vi "Calibrate VNA.vi"(8 "error in (no error)":errorcluster, 9 "Cal kit type":enum16{"E-CAL", "Mechanical"}(ring), 10 "Calibration mode":enum16{"1 Port", "2  Port", "3 Port", "4 Port"}(ring), 11 "VNA-PNA in":refnum<class "VNA-PNA.lvclass">) -> (0 "error out":errorcluster, 3 "VNA-PNA out":refnum<class "VNA-PNA.lvclass">)   [LabVIEW 2020, in "VNA-PNA.lvclass"]
uses:
  VNA-PNA.lvclass
  C:/Sandbox/Git_Sandbox/WiSpry Test Framework source code (LV20)/WiSpry Test Framework/Instruments/Instrument.lvclass
  C:/Sandbox/Git_Sandbox/WiSpry Test Framework source code (LV20)/WiSpry Test Framework/Instruments/Vector Network Analyzer/Vector Network Analyzer.lvclass
  Vector Network Analyzer.lvclass/Vector Network Analyzer.ctl
  Instrument.lvclass/Instrument.ctl
  Instrument.lvclass
  Vector Network Analyzer.lvclass
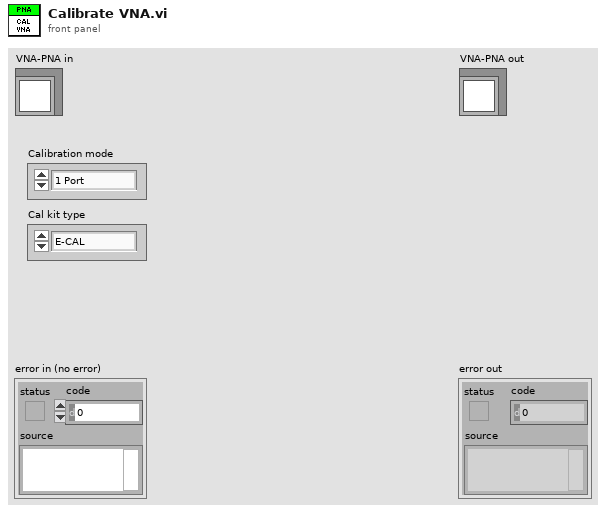
[diagram p1: front panel]
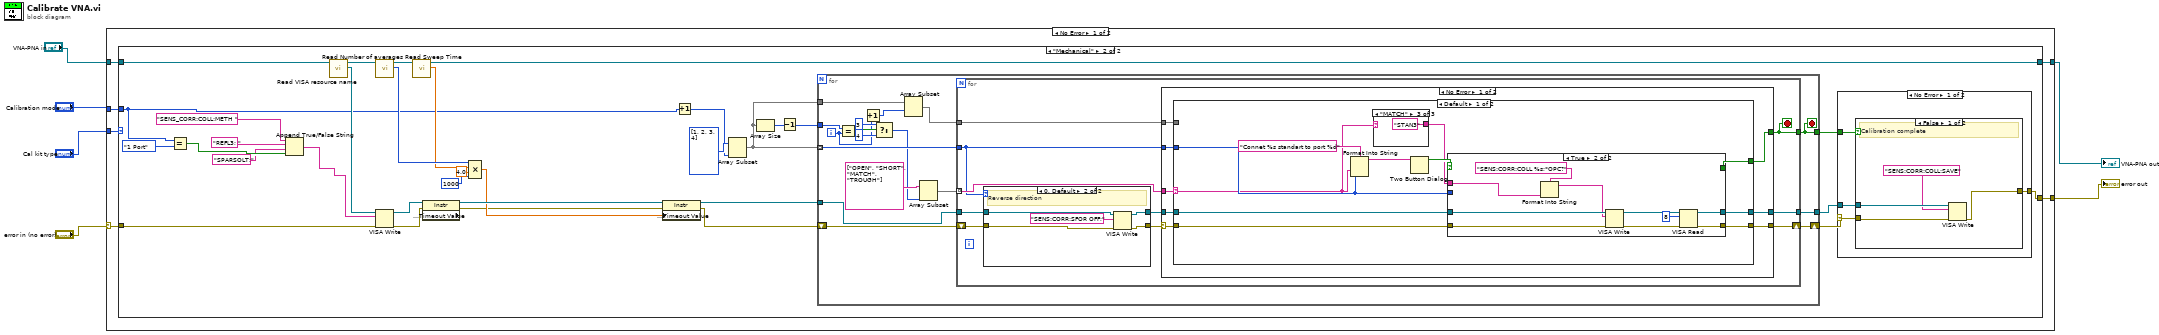
[diagram p0: block diagram]
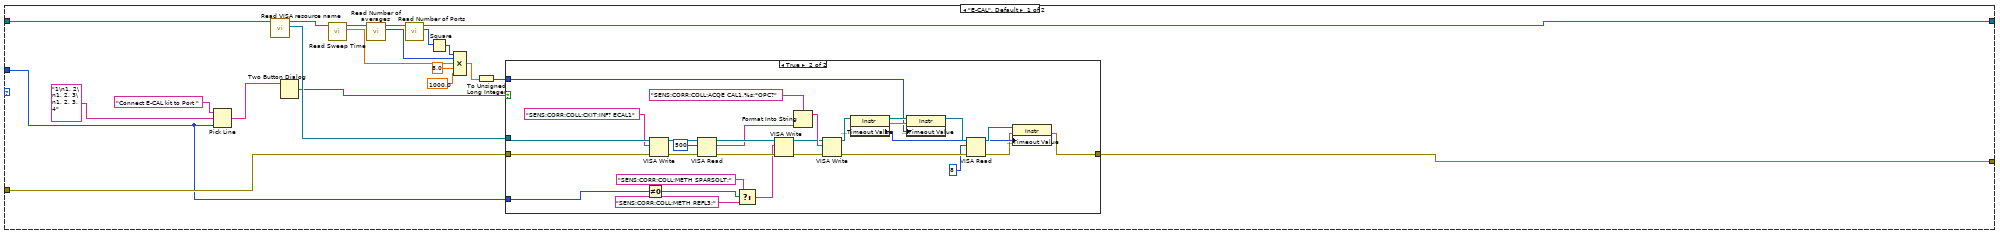
[diagram p2: hidden frame]
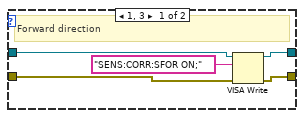
[diagram p6: hidden frame]
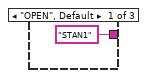
[diagram p7: hidden frame]
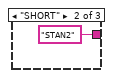
[diagram p8: hidden frame]
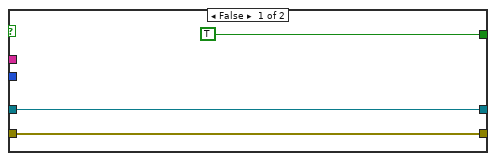
[diagram p9: hidden frame]
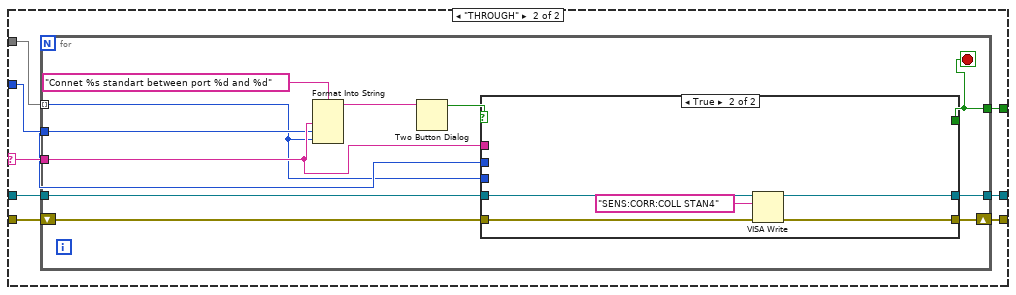
[diagram p10: hidden frame]
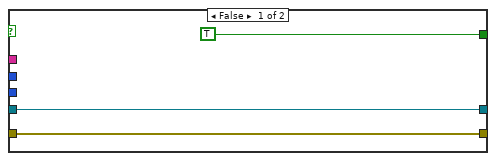
[diagram p11: hidden frame]
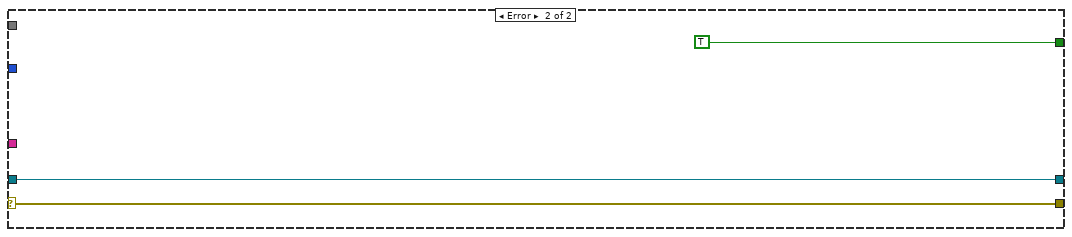
[diagram p12: hidden frame]
diagram:
  n1 = case shown="No Error" "error in (no error)" {
    selector: "error in (no error)" -> [w10 w209]
    tunnel: "Calibration mode" -> [w12 _]
    tunnel: "VNA-PNA in" -> [w11 w210]
    tunnel: [w9 w209] -> w3
    tunnel: [w8 w210] -> w2
    tunnel: "Cal kit type" -> [w7 _]
    frame No Error {
      n2 = case shown="\"Mechanical\"" w7 {
        tunnel: w12 -> [w13 w66]
        tunnel: w11 -> [w33 w91]
        tunnel: w10 -> [w31 w92]
        tunnel: [w30 w67] -> w9
        tunnel: [w23 w73] -> w8
        frame "E-CAL", Default {
          n3 = Pick Line(string ("")="Connect E-CAL kit to Port " ("message"), multi-line string="1\n1, 2\n1, 2, 3\n1, 2, 3, 4", line index=w13) -> (output string=w26:string)
          n4 = call "Read VISA resource name.vi"("Instrument in"=w33) -> ("VISA resource name"=w32:refnum<visa-resource-name>, "Instrument out"=w25:refnum<class "VNA-PNA.lvclass">)  [unwired: 9 in]
          n5 = Two Button Dialog(message=w26) -> (T button?=w29:bool)  [unwired: 2 in]
          n6 = call "Read Sweep Time.vi"("Vector Network Analyzer in"=w25) -> ("Sweep Time"=w18:dbl, "Vector Network Analyzer out"=w24:refnum<class "VNA-PNA.lvclass">)  [unwired: 9 in]
          n7 = call "Read Number of averages.vi"("Vector Network Analyzer in"=w24) -> ("Number of averages"=w19:i32, "Vector Network Analyzer out"=w22:refnum<class "VNA-PNA.lvclass">)  [unwired: 9 in]
          n8 = call "Read Number of Ports.vi"("Vector Network Analyzer in"=w22) -> ("Number of Ports"=w21:i32, "Vector Network Analyzer out"=w23:refnum<class "VNA-PNA.lvclass">)  [unwired: 9 in]
          n9 = Square(x=w21) -> (x^2=w20:i32)
          n10 = Compound Arithmetic op=MULTIPLY(w20, w19, w18, 8.0 ("value"), 1000.0 ("value")) -> (w15:dbl)
          n11 = To Unsigned Long Integer(number=w15) -> (unsigned 32bit integer=w14:u32)
          n12 = case shown="True" w29 {
            tunnel: w32 -> [_ w51]
            tunnel: w31 -> [w34 w52]
            tunnel: [w34 w53] -> w30
            tunnel: w14 -> [_ w54]
            tunnel: w13 -> [_ w44]
            frame False {
            }
            frame True {
              n13 = Not Equal To 0?(x=w44) -> (x != 0?=w43:bool)
              n14 = VISA Write(VISA resource name=w51, write buffer="SENS:CORR:COLL:CKIT:INF? ECAL1", error in (no error)=w52) -> (VISA resource name out=w48:refnum<visa-resource-name>, error out=w49:errorcluster)  [unwired: 1 out]
              n15 = VISA Read(VISA resource name=w48, byte count=u32 500, error in (no error)=w49) -> (VISA resource name out=w46:refnum<visa-resource-name>, read buffer=w38:string, error out=w45:errorcluster)  [unwired: 1 out]
              n16 = Select(t="SENS:CORR:COLL:METH SPARSOLT;" ("write buffer"), s=w43, f="SENS:CORR:COLL:METH REFL3;") -> (s? t:f=w41:string)
              n17 = VISA Write(VISA resource name=w46, write buffer=w41, error in (no error)=w45) -> (VISA resource name out=w36:refnum<visa-resource-name>, error out=w35:errorcluster)  [unwired: 1 out]
              n18 = Format Into String(format string="SENS:CORR:COLL:ACQE CAL1,%s;*OPC?", w38) -> (resulting string=w37:string)  [unwired: 2 in, 1 out]
              n19 = VISA Write(VISA resource name=w36, write buffer=w37, error in (no error)=w35) -> (VISA resource name out=w63:refnum<visa-resource-name>, error out=w59:errorcluster)  [unwired: 1 out]
              n20 = property class="Instr"(reference=w63) -> (reference out=w62:refnum<visa-resource-name>, error out=w61:errorcluster, "General Settings:Timeout Value"=w56:u32)  [unwired: 1 in]
              n21 = property class="Instr"(reference=w62, error in=w61, "General Settings:Timeout Value"=w54) -> (reference out=w60:refnum<visa-resource-name>)  [unwired: 1 out]
              n22 = VISA Read(VISA resource name=w60, byte count=u32 8, error in (no error)=w59) -> (VISA resource name out=w57:refnum<visa-resource-name>, error out=w55:errorcluster)  [unwired: 2 out]
              n23 = property class="Instr"(reference=w57, error in=w55, "General Settings:Timeout Value"=w56) -> (error out=w53:errorcluster)  [unwired: 1 out]
            }
          }
        }
        frame "Mechanical" {
          n24 = Equal?(x=w66, y=enum16{"1 Port", "2  Port", "3 Port", "4 Port"}."1 Port") -> (x = y?=w95:bool)
          n25 = Append True/False String(1:w95, 2:"SPARSOLT;", 3:"REFL3; ", 4:"SENS_CORR:COLL:METH ") -> (0:w65:string)
          n26 = call "Read VISA resource name.vi"("Instrument in"=w91) -> ("VISA resource name"=w90:refnum<visa-resource-name>, "Instrument out"=w85:refnum<class "VNA-PNA.lvclass">)  [unwired: 9 in]
          n27 = call "Read Number of averages.vi"("Vector Network Analyzer in"=w85) -> ("Number of averages"=w83:i32, "Vector Network Analyzer out"=w84:refnum<class "VNA-PNA.lvclass">)  [unwired: 9 in]
          n28 = VISA Write(VISA resource name=w90, write buffer=w65, error in (no error)=w92) -> (VISA resource name out=w81:refnum<visa-resource-name>, error out=w80:errorcluster)  [unwired: 1 out]
          n29 = call "Read Sweep Time.vi"("Vector Network Analyzer in"=w84) -> ("Sweep Time"=w82:dbl, "Vector Network Analyzer out"=w73:refnum<class "VNA-PNA.lvclass">)  [unwired: 9 in]
          n30 = property class="Instr" props=["General Settings:Timeout Value"](reference=w81, error in=w80) -> (reference out=w79:refnum<visa-resource-name>, error out=w76:errorcluster)  [unwired: 1 out]
          n31 = Compound Arithmetic op=MULTIPLY(w83, w82, 4.0 ("value"), 1000 ("value")) -> (w77:dbl)
          n32 = property class="Instr"(reference=w79, error in=w76, "General Settings:Timeout Value"=w77) -> (reference out=w75:refnum<visa-resource-name>, error out=w74:errorcluster)
          n33 = Increment(x=w66) -> (x+1=w88:enum16{"1 Port", "2  Port", "3 Port", "4 Port"})
          n34 = Array Subset(array=i32[] [1, 2, 3, 4], length=w88) -> (w71:i32[])  [unwired: 1 in]
          n35 = Array Size(array=w71) -> (size(s)=w87:i32)
          n36 = Decrement(x=w87) -> (x-1=w86:i32)
          n37 = for {
            shift-right: [w109] -> w70
            shift-left: w74 -> [w117]
            tunnel: w71 -> [w116] mode=indexing
            tunnel: w86 -> [w123]
            tunnel: w75 -> [w115]
            tunnel: w71 -> [w113]
            tunnel: [w108] -> w69
            tunnel: [w107] -> w68
            i -> [w111]
            stop <- w108 stop-if-true
            n38 = Equal?(x=w123, y=w111) -> (x = y?=w121:bool)
            n39 = Increment(x=w111) -> (x+1=w112:i32)
            n40 = Select(t=3, s=w121, f=4) -> (s? t:f=w114:i32)
            n41 = Array Subset(array=w113, index=w112) -> (w110:i32[])  [unwired: 1 in]
            n42 = Array Subset(array=string[] ["OPEN", "SHORT", "MATCH", "TROUGH"], length=w114) -> (w118:string[])  [unwired: 1 in]
            n43 = for {
              tunnel: w118 -> [w132] mode=indexing
              shift-right: [w131] -> w109
              shift-left: w117 -> [w127]
              tunnel: [w133] -> w108
              tunnel: w115 -> [w124]
              tunnel: w116 -> [w128]
              tunnel: w110 -> [w130]
              tunnel: [w129] -> w107
              stop <- w133 stop-if-true
              n44 = case shown="0, Default" w128 {
                tunnel: w127 -> [w135 w140]
                tunnel: [w138 w143] -> w126
                tunnel: [w137 w142] -> w125
                tunnel: w124 -> [w136 w141]
                frame 1, 3 {
                  # "Forward direction"
                  n45 = VISA Write(VISA resource name=w136, write buffer="SENS:CORR:SFOR ON;", error in (no error)=w135) -> (VISA resource name out=w137:refnum<visa-resource-name>, error out=w138:errorcluster)  [unwired: 1 out]
                }
                frame 0, Default {
                  # "Reverse direction"
                  n46 = VISA Write(VISA resource name=w141, write buffer="SENS:CORR:SFOR OFF;", error in (no error)=w140) -> (VISA resource name out=w142:refnum<visa-resource-name>, error out=w143:errorcluster)  [unwired: 1 out]
                }
              }
              n47 = case shown="No Error" w126 {
                selector: w126 -> [w150 w207]
                tunnel: [w147 TRUE] -> w133
                tunnel: w132 -> [w151 _]
                tunnel: w125 -> [w148 w206]
                tunnel: w128 -> [w149 _]
                tunnel: [w146 w207] -> w131
                tunnel: w130 -> [w145 _]
                tunnel: [w144 w206] -> w129
                frame No Error {
                  n48 = case shown="Default" w151 {
                    selector: w151 -> [w153 w184]
                    tunnel: w150 -> [w159 w186]
                    tunnel: w149 -> [w157 w181]
                    tunnel: w148 -> [w158 w185]
                    tunnel: [w156 w183] -> w147
                    tunnel: [w155 w182] -> w146
                    tunnel: w145 -> [_ w180]
                    tunnel: [w154 w179] -> w144
                    frame Default {
                      n49 = Format Into String(format string="Connet %s standart to port %d", w153, w157) -> (resulting string=w161:string)  [unwired: 2 in, 1 out]
                      n50 = case shown="\"MATCH\"" w153 {
                        tunnel: ["STAN1" "STAN2" "STAN3"] -> w152
                        frame "OPEN", Default {
                        }
                        frame "SHORT" {
                        }
                        frame "MATCH" {
                        }
                      }
                      n51 = Two Button Dialog(message=w161) -> (T button?=w160:bool)  [unwired: 2 in]
                      n52 = case shown="True" w160 {
                        tunnel: w159 -> [w167 w176]
                        tunnel: w158 -> [w166 w175]
                        tunnel: w152 -> [_ w177]
                        tunnel: w157 -> [_ _]
                        tunnel: [TRUE _] -> w156
                        tunnel: [w167 w171] -> w155
                        tunnel: [w166 w170] -> w154
                        frame False {
                        }
                        frame True {
                          n53 = Format Into String(format string="SENS:CORR:COLL %s;*OPC?", w177) -> (resulting string=w174:string)  [unwired: 2 in, 1 out]
                          n54 = VISA Write(VISA resource name=w175, write buffer=w174, error in (no error)=w176) -> (VISA resource name out=w173:refnum<visa-resource-name>, error out=w172:errorcluster)  [unwired: 1 out]
                          n55 = VISA Read(VISA resource name=w173, byte count=u32 8, error in (no error)=w172) -> (VISA resource name out=w170:refnum<visa-resource-name>, error out=w171:errorcluster)  [unwired: 2 out]
                        }
                      }
                    }
                    frame "THROUGH" {
                      n56 = for {
                        tunnel: w185 -> [w193]
                        tunnel: w184 -> [w192]
                        tunnel: [w189] -> w183
                        tunnel: w181 -> [w190]
                        shift-right: [w191] -> w182
                        shift-left: w186 -> [w194]
                        tunnel: w180 -> [w188] mode=indexing
                        tunnel: [w187] -> w179
                        stop <- w189 stop-if-true
                        n57 = Format Into String(format string="Connet %s standart between port %d and %d", w192, w190, w188) -> (resulting string=w196:string)  [unwired: 2 in, 1 out]
                        n58 = Two Button Dialog(message=w196) -> (T button?=w195:bool)  [unwired: 2 in]
                        n59 = case shown="True" w195 {
                          tunnel: w194 -> [w199 w205]
                          tunnel: w193 -> [w198 w204]
                          tunnel: w192 -> [_ _]
                          tunnel: w190 -> [_ _]
                          tunnel: [TRUE _] -> w189
                          tunnel: [w199 w203] -> w191
                          tunnel: w188 -> [_ _]
                          tunnel: [w198 w202] -> w187
                          frame False {
                          }
                          frame True {
                            n60 = VISA Write(VISA resource name=w204, write buffer="SENS:CORR:COLL STAN4", error in (no error)=w205) -> (VISA resource name out=w202:refnum<visa-resource-name>, error out=w203:errorcluster)  [unwired: 1 out]
                          }
                        }
                      }
                    }
                  }
                }
                frame Error {
                }
              }
            }
          }
          n61 = case shown="No Error" w70 {
            selector: w70 -> [w99 w106]
            tunnel: w69 -> [w100 _]
            tunnel: w68 -> [w98 _]
            tunnel: [w97 w106] -> w67
            frame No Error {
              n62 = case shown="False" w100 {
                tunnel: w99 -> [w104 w105]
                tunnel: w98 -> [w103 _]
                tunnel: [w102 w105] -> w97
                frame False {
                  # "Calibration complete"
                  n63 = VISA Write(VISA resource name=w103, write buffer="SENS:CORR:COLL:SAVE", error in (no error)=w104) -> (error out=w102:errorcluster)  [unwired: 2 out]
                }
                frame True {
                }
              }
            }
            frame Error {
            }
          }
        }
      }
    }
    frame Error {
    }
  }
  "error out" <- w3
  "VNA-PNA out" <- w2
